vi "Map Function (SubVI).vi"(7 "x-input":dbl, 8 "y max":dbl, 9 "y min":dbl, 10 "x max":dbl, 11 "x min":dbl) -> (3 "y-output":dbl)   [LabVIEW 2017]
panel:
  out "c":dbl
  out "m":dbl
  # "This subVI performs the 'map' functionality, analogous to the map() function on Arduino.\n\nIt takes in x-min and x-max and map them to y-min and y-max."
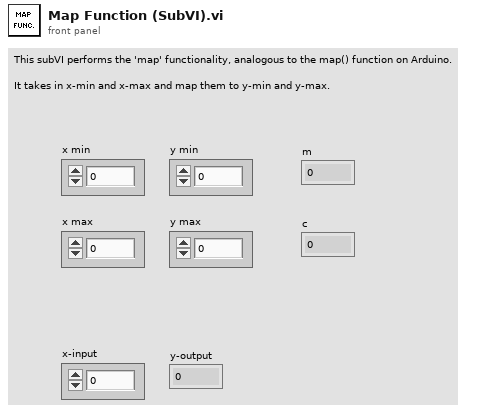
[diagram p1: front panel]
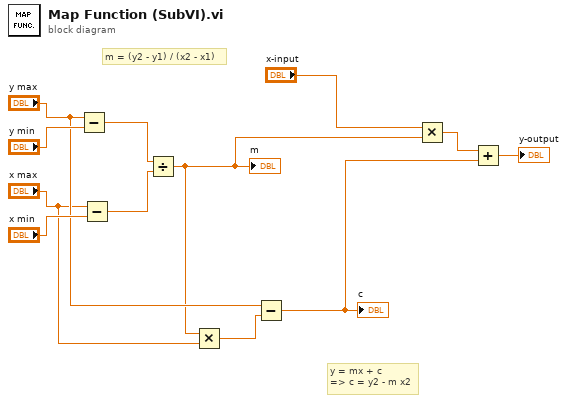
[diagram p0: block diagram]
diagram:
  # "y = mx + c\n=> c = y2 - m x2"
  # "m = (y2 - y1) / (x2 - x1)"
  n1 = Subtract(x="y max", y="y min") -> (x-y=w10:dbl)
  n2 = Subtract(x="x max", y="x min") -> (x-y=w9:dbl)
  n3 = Divide(x=w10, y=w9) -> (x/y=w4:dbl)
  "m" <- w4
  n4 = Multiply(x=w4, y="x max") -> (x*y=w6:dbl)
  n5 = Subtract(x="y max", y=w6) -> (x-y=w2:dbl)
  "c" <- w2
  n6 = Multiply(x="x-input", y=w4) -> (x*y=w3:dbl)
  n7 = Add(x=w3, y=w2) -> (x+y=→"y-output":dbl)
